vi "e.gate Example - HighSpeedPort e.con Archive.vi"(8 "Fehler (Eingang, kein Fehler)":errorcluster, 11 "IP Address":string="IP Address") -> (0 "Fehler (Ausgang)":errorcluster)   [LabVIEW 2016]
uses:
  e.gate Protocol Type.ctl
  e.gate Decode UDBF - Stream.vi
panel:
  out "Signalverlaufsdiagramm":dbl[](graph)
  in  "Channel":i32
  in  "Stopp":bool
  # "Example - HighSpeedPort - e.con Archive"
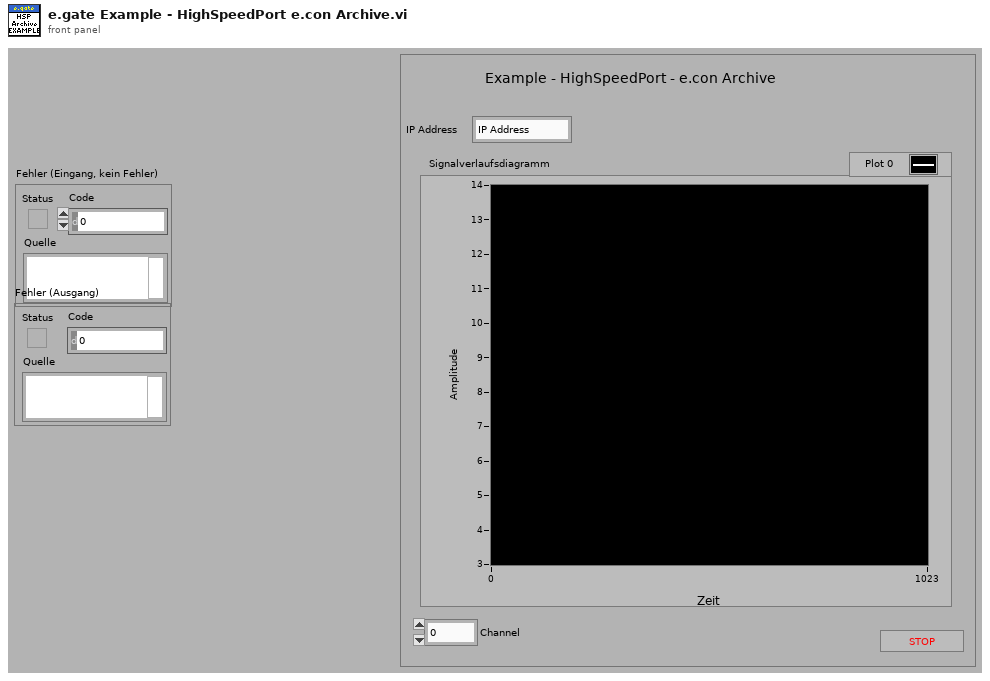
[diagram p1: front panel]
types:
  T1 = typedef "e.gate Protocol Type.ctl" = enum16{"ASCII", "HighspeedPort Online", "HighspeedPort Buffer", "eGateHighspeedPortDLL "}
  T2 = typedef "e.gate Configuration.ctl" = cluster{"connection ID":refnum<k5>, "IPAddress":string, "BufferIndex":i32, "StateMessage":string, "StateCode":i8, "HeaderSize":i32, "BufferSize":i32, "IsBigEndian":i32, "Version":i32, "ChannelCount":i32, "FrameLength":i32, "StartTime":dbl, "dActTimeToSecondFactor":dbl, "StartTimeToDayFactor":dbl, "BufferFillRate":dbl, "SampleRate":dbl, "ChannelData":T3[], "DecodeTimeFormat":string, "SummaryPath":string, "WithCheckSum":i32, "dActTimeDataType":T4, "MaxWriteCount":i32, "MaxReadCount":i32, "TempOffsetRead":i32, "TempLengthRead":i32, "Protocol":T1, "IsSupported":i32, "InputAccessList":i32[], "OutputAccessList":i32[], "DataSource":enum16{"CircleBuffer", "test.con Logger", "test.con Archive"}, "Modules":T5[], "DLL-Handle":T6}
  T3 = typedef "e.gate Channel Data.ctl" = cluster{"VariableName":string, "DataDirection":string, "DataType":string, "DataTypeIndex":T4, "Precision":i16, "FieldLengtht":i16, "ByteCount":i32, "Format":string, "Unit":string, "InputAccessOffset":i32, "OutputAccessOffset":i16, "InputAccessIndex":i16, "OutputAccessIndex":i16, "VarType":string}
  T4 = typedef "e.gate Data Type.ctl" = enum16{"NO", "BOOL", "SINT8", "USINT8", "SINT16", "USINT16", "SINT32", "USINT32", "FLOAT", "SET8", "SET16", "SET32", "DOUBLE", "SINT64", "USINT64", "SET64"}
  T5 = typedef "e.gate Module  Data.ctl" = cluster{"Type":string, "Location":string, "VariablesCount":i16, "UartIndex":i16, "Address":i16, "SystemOffset":i16}
  T6 = typedef "e.gateHSP_DLLhandle.ctl" = cluster{"clientInstance":i32, "connectionInstance":i32}
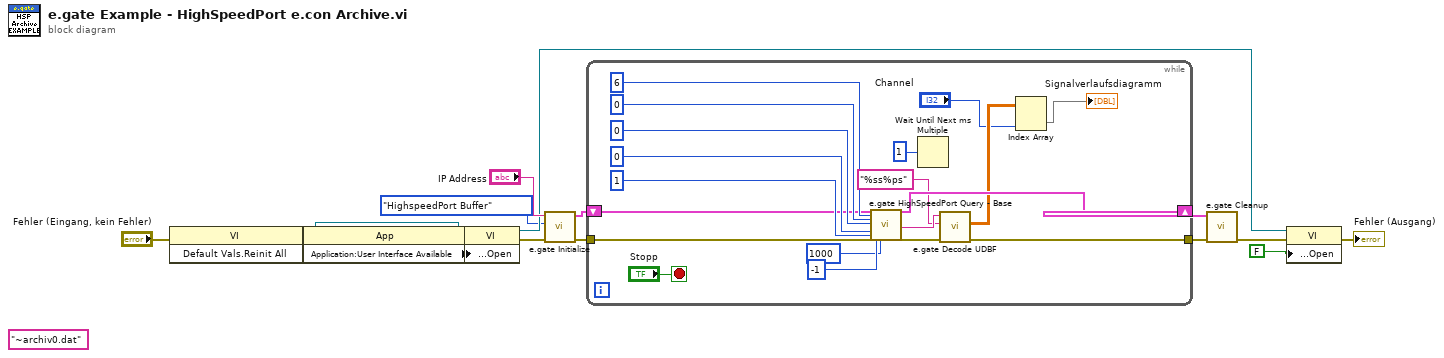
[diagram p0: block diagram]
diagram:
  (unwired) "~archiv0.dat" ("File or relative Path")
  n1 = invoke class="VI" method="Default Vals.Reinit All"(error in="Fehler (Eingang, kein Fehler)") -> (reference out=w13:refnum<vi>, error out=w11:errorcluster)  [unwired: 2 in, 1 out]
  n2 = property class="App"(error in=w11) -> (error out=w10:errorcluster, "Application:User Interface Available"=w12:bool)  [unwired: 1 in, 1 out]
  n3 = property class="VI"(reference=w13, error in=w10, "Front Panel.Open"=w12) -> (reference out=w5:refnum<vi>, error out=w8:errorcluster)
  n4 = call "e.gate Initialize.vi"("error in (no error)"=w8, "Protocol"=e.gate_Protocol_Type."HighspeedPort Buffer", "IP Address"="IP Address") -> ("error out"=w15:errorcluster, "e.gate Configuration"=w16:T2)  [unwired: 1 in, 6 out]
  n5 = while {
    tunnel: w15 -> [w22]
    tunnel: [w31] -> w2
    shift-right: [w29] -> w1
    shift-left: w16 -> [w23]
    stop <- "Stopp" stop-if-true
    n6 = call "e.gate HighSpeedPort Query - Base.vi"("e.gate Configuration in"=w23, "Command"=6, "OffsetWrite"=0, "LengthWrite"=0, "OffsetRead"=0, "LengthRead"=1, "error in (no error)"=w22, "TCP LengthReadt"=-1, "Timeout (1000)"=1000) -> ("e.gate Configuration out"=w29:T2, "data out (string)"=w30:string, "error out"=w32:errorcluster)  [unwired: 1 in, 15 out]
    n7 = Wait Until Next ms Multiple(millisecond multiple=u32 1 ("Vielfache von ms")) -> ()  [unwired: 1 out]
    n8 = call-poly "e.gate Decode UDBF.vi"("error in (no error)"=w32, "DecodeTimeFormat"="%ss%ps", "UDBF Stream"=w30) -> ("error out"=w31:errorcluster, "data array (double)"=w19:dbl[][])  [unwired: 7 out]
    n9 = Index Array(array=w19, index (col)="Channel") -> (element=→"Signalverlaufsdiagramm":dbl[])  [unwired: 1 in]
  }
  n10 = call "e.gate Cleanup.vi"("error in (no error)"=w2, "e.gate Configuration"=w1) -> ("error out"=w7:errorcluster)  [unwired: 9 out]
  n11 = property class="VI"(reference=w5, error in=w7, "Front Panel.Open"=FALSE ("Frontpanel-Fenster:Öffnen")) -> (error out=→"Fehler (Ausgang)":errorcluster)  [unwired: 1 out]
